vi "benchmarks_largeBinaryMD5.vi"() -> ()   [LabVIEW 2013]
uses:
  MD5/MD5.lvclass
  <vilib>/Analysis/baseanly.llb/Mean (DBL).vi
  MD5/MD5.lvlib
  <vilib>/Analysis/NI_AALBase.lvlib
panel:
  out "% gain":dbl
  out "LVOS":u8[](array[numeric]) format="%.0x"
  out "NI":string
  out "LVOS":dbl
  out "NI":dbl
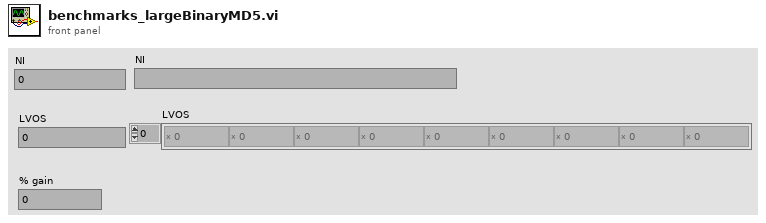
[diagram p1: front panel]
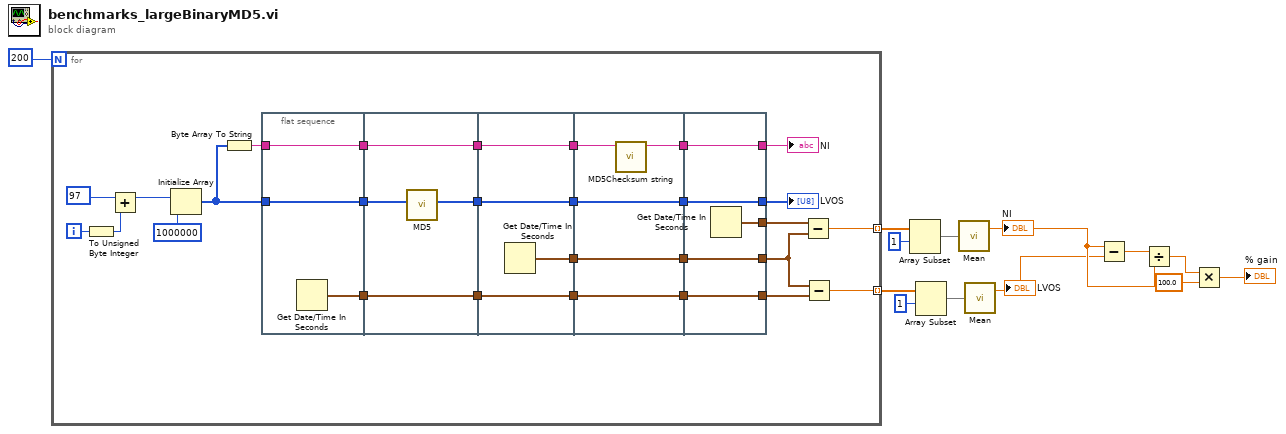
[diagram p0: block diagram]
diagram:
  n1 = for {
    N: 200 -> [_]
    tunnel: [w27] -> w12 mode=indexing
    tunnel: [w26] -> w7 mode=indexing
    i -> [w16]
    n2 = To Unsigned Byte Integer(number=w16) -> (unsigned 8bit integer=w17:u8)
    n3 = Add(x=u8 97 ("Numeric"), y=w17) -> (x+y=w18:u8)
    n4 = Initialize Array(w18, 1000000 ("dimension size")) -> (w23:u8[])
    n5 = Byte Array To String(unsigned byte array=w23) -> (string=w24:string)
    n6 = flat-sequence {
      tunnel: [w44] -> w41
      tunnel: w23 -> [w43]
      tunnel: [w43] -> w40
      tunnel: w24 -> [w42]
      tunnel: [w42] -> w39
      tunnel: w41 -> [w48]
      tunnel: [w48] -> w38
      tunnel: [w46] -> w37
      tunnel: w40 -> [w47]
      tunnel: w39 -> [w45]
      tunnel: [w45] -> w36
      tunnel: [w52] -> w35
      tunnel: [w51] -> w34
      tunnel: w38 -> [w51]
      tunnel: [w50] -> w33
      tunnel: w37 -> [w50]
      tunnel: w36 -> [w49]
      tunnel: [w49] -> w32
      tunnel: [w57] -> w31
      tunnel: w35 -> [w57]
      tunnel: [w56] -> w30
      tunnel: w34 -> [w56]
      tunnel: [w54] -> w29
      tunnel: [w55] -> w28
      tunnel: w33 -> [w55]
      tunnel: w32 -> [w53]
      tunnel: [w62] -> w21
      tunnel: w31 -> [w62]
      tunnel: [w61] -> w20
      tunnel: w30 -> [w61]
      tunnel: [w60] -> w22
      tunnel: [w59] -> w15
      tunnel: w29 -> [w59]
      tunnel: [w58] -> w14
      tunnel: w28 -> [w58]
      frame #0 {
        n7 = Get Date/Time In Seconds() -> (seconds since 1Jan1904=w44:timestamp)
      }
      frame #1 {
        n8 = call "MD5.vi"("data"=w47) -> ("MD5 hash"=w46:u8[])  [unwired: 10 in]
      }
      frame #2 {
        n9 = Get Date/Time In Seconds() -> (seconds since 1Jan1904=w52:timestamp)
      }
      frame #3 {
        n10 = call <vilib>:"MD5Checksum string.vi"("Message String"=w53) -> ("MD5 message-digest"=w54:string)  [unwired: 10 in]
      }
      frame #4 {
        n11 = Get Date/Time In Seconds() -> (seconds since 1Jan1904=w60:timestamp)
      }
    }
    n12 = Subtract(x=w22, y=w21) -> (x-y=w27:dbl)
    n13 = Subtract(x=w21, y=w20) -> (x-y=w26:dbl)
    "NI" <- w15
    "LVOS" <- w14
  }
  n14 = Array Subset(array=w12, index=1) -> (w10:dbl[])  [unwired: 1 in]
  n15 = Array Subset(array=w7, index=1) -> (w9:dbl[])  [unwired: 1 in]
  n16 = call-poly <vilib>:"Mean.vi"("X"=w10) -> ("mean"=w2:dbl)  [unwired: 1 out]
  "NI" <- w2
  n17 = call-poly <vilib>:"Mean.vi"("X"=w9) -> ("mean"=w1:dbl)  [unwired: 1 out]
  "LVOS" <- w1
  n18 = Subtract(x=w2, y=w1) -> (x-y=w6:dbl)
  n19 = Divide(x=w6, y=w2) -> (x/y=w4:dbl)
  n20 = Multiply(x=w4, y=100.0) -> (x*y=→"% gain":dbl)
